vi "stopShooting.vi"(8 "error in (no error)":errorcluster, 10 "stop":bool, 11 "CameraController in":refnum<class "CameraController.lvclass">) -> (0 "error out":errorcluster, 1 "Stopped":bool=TRUE, 2 "Array":path[](array[path]), 3 "CameraController out":refnum<class "CameraController.lvclass">)   [LabVIEW 2011, in "Hardware.lvlib" / "Channels.lvlib" / "CameraController.lvclass"]
uses:
  CameraController.lvclass
  CameraAcquisitor.lvclass
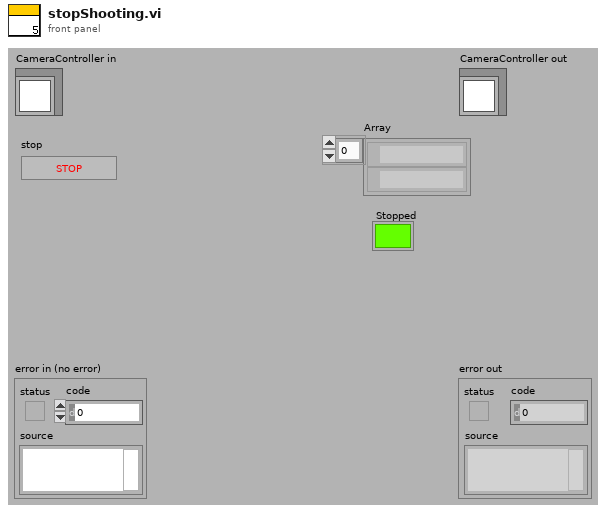
[diagram p1: front panel]
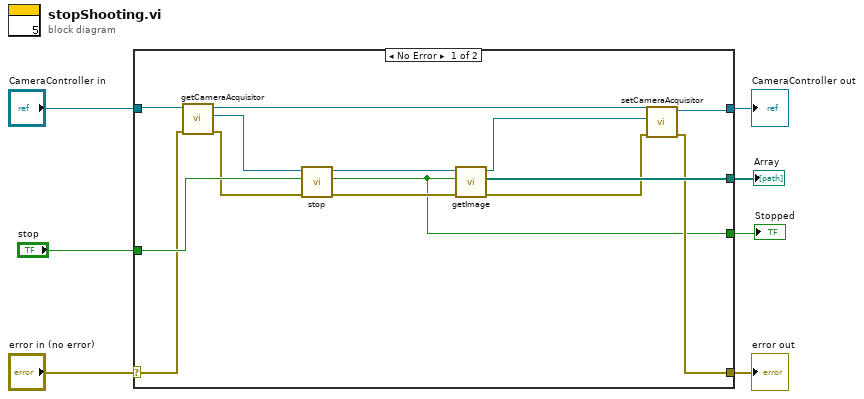
[diagram p0: block diagram]
diagram:
  n1 = case shown="No Error" "error in (no error)" {
    selector: "error in (no error)" -> [w17 w23]
    tunnel: [w9 w23] -> w6
    tunnel: [w14 w22] -> w4
    tunnel: "CameraController in" -> [w18 w22]
    tunnel: "stop" -> [w19 _]
    tunnel: [w8 _] -> w2
    tunnel: [w12 _] -> w1
    frame No Error {
      n2 = call-dynamic "getCameraAcquisitor.vi"("error in (no error)"=w17, "CameraController.lvclass in"=w18) -> ("error out"=w16:errorcluster, "CameraAcquisitor.lvclass"=w15:refnum<class "CameraAcquisitor.lvclass">, "CameraController.lvclass out"=w13:refnum<class "CameraController.lvclass">)  [unwired: 7 in]
      n3 = call-dynamic "stop.vi"("error in (no error)"=w16, "Stop"=w19, "CameraAcquisitor in"=w15) -> ("error out"=w20:errorcluster, "Stopped"=w8:bool, "CameraAcquisitor out"=w21:refnum<class "CameraAcquisitor.lvclass">)  [unwired: 6 in]
      n4 = call-dynamic "getImage.vi"("error in (no error)"=w20, "stop"=w8, "CameraAcquisitor in"=w21) -> ("error out"=w10:errorcluster, "Array"=w12:path[], "CameraAcquisitor out"=w11:refnum<class "CameraAcquisitor.lvclass">)  [unwired: 6 in]
      n5 = call-dynamic "setCameraAcquisitor.vi"("error in (no error)"=w10, "Hardware:Channels.lvlib:CameraAcquisitor.lvclass"=w11, "CameraController.lvclass in"=w13) -> ("error out"=w9:errorcluster, "CameraController.lvclass out"=w14:refnum<class "CameraController.lvclass">)  [unwired: 7 in]
    }
    frame Error {
    }
  }
  "error out" <- w6
  "CameraController out" <- w4
  "Stopped" <- w2
  "Array" <- w1
